vi "Camera Viewing Test.vi"() -> ()   [LabVIEW 2018]
uses:
  Classes/Realsense Cam/Private/Stream Config STYP.ctl
  Classes/Realsense Cam/Private/Stream Types Enum STYP.ctl
  Classes/Video Cam Processor/Video Cam Processor.lvclass
  C:/Users/aaron.jencks/Documents/GitHub/emerson_seed_object_detection/LabVIEW/Projects/Paul's Video Viewer/Classes/Realsense Cam Video File Wrapper/Realsense Cam File Wrapper.lvclass
  Classes/Realsense Cam/Realsense Cam.lvclass
panel:
  out "Roughness (inches)":T1
  out "spreadsheet string":string
  in  "Data Collection Interval (ms)":u32=10000
  in  "Next":bool
  out "Roughness":T1
  in  "Segmentedness":i32=10
  out "Image":T2(plugin-control)
  in  "stop":bool
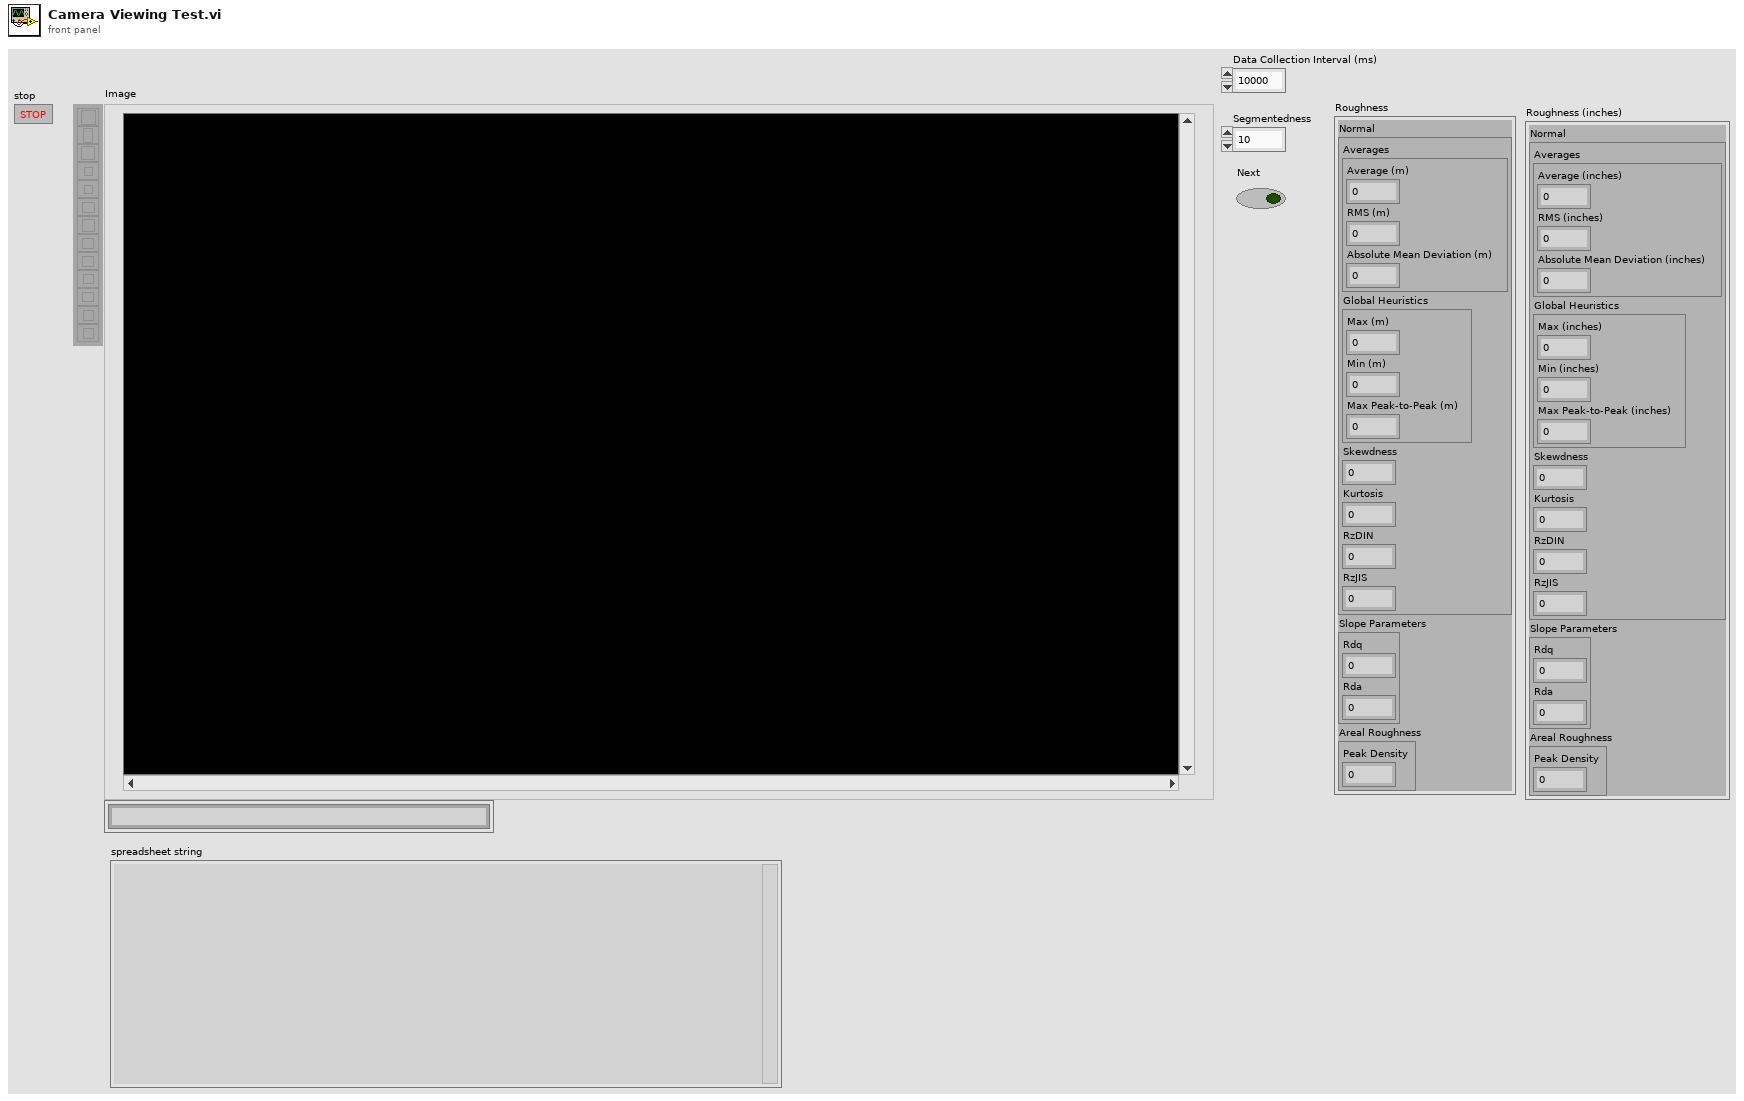
[diagram p1: front panel]
types:
  T1 = cluster{"Normal":cluster{"Averages":cluster{"Average":dbl, "RMS":dbl, "Absolute Mean Deviation":dbl}, "Global Heuristics":cluster{"Max":dbl, "Min":dbl, "Max Peak-to-Peak":dbl}, "Skewdness":dbl, "Kurtosis":dbl, "RzDIN":dbl, "RzJIS":dbl}, "Slope Parameters":cluster{"Rdq":dbl, "Rda":dbl}, "Areal Roughness":cluster{"Peak Density":dbl}}
  T2 = typedef "IMAQ Image.ctl" = refnum<image>
  T3 = cluster{"Normal":cluster{"Averages":cluster{"Average":dbl, "RMS":dbl, "Absolute Mean Deviation":dbl}, "Global Heuristics":cluster{"Max":dbl, "Min":dbl, "Max Peak-to-Peak":dbl}, "Skewdness":dbl, "Kurtosis":dbl, "RzDIN":dbl, "RzJIS":dbl}, "Slope Parameters":cluster{"Rdq":dbl, "Rda":dbl}, "Areal Roughness":cluster{"Peak Density":dbl}}[]
  T4 = typedef "Image Type" = u32
  T5 = typedef "Realsense Cam.lvclass/Stream Config STYP.ctl" = cluster{"Stream Type":T6, "Resolution":u16}
  T6 = typedef "Realsense Cam.lvclass/Stream Types Enum STYP.ctl" = enum16{"Depth", "Left IR", "Left IR Unrectified", "Right IR", "Right IR Unrectified", "Color", "RGB Ext."}
  T7 = cluster{"Average":dbl, "RMS":dbl, "Absolute Mean Deviation":dbl}
  T8 = cluster{"Max":dbl, "Min":dbl, "Max Peak-to-Peak":dbl}
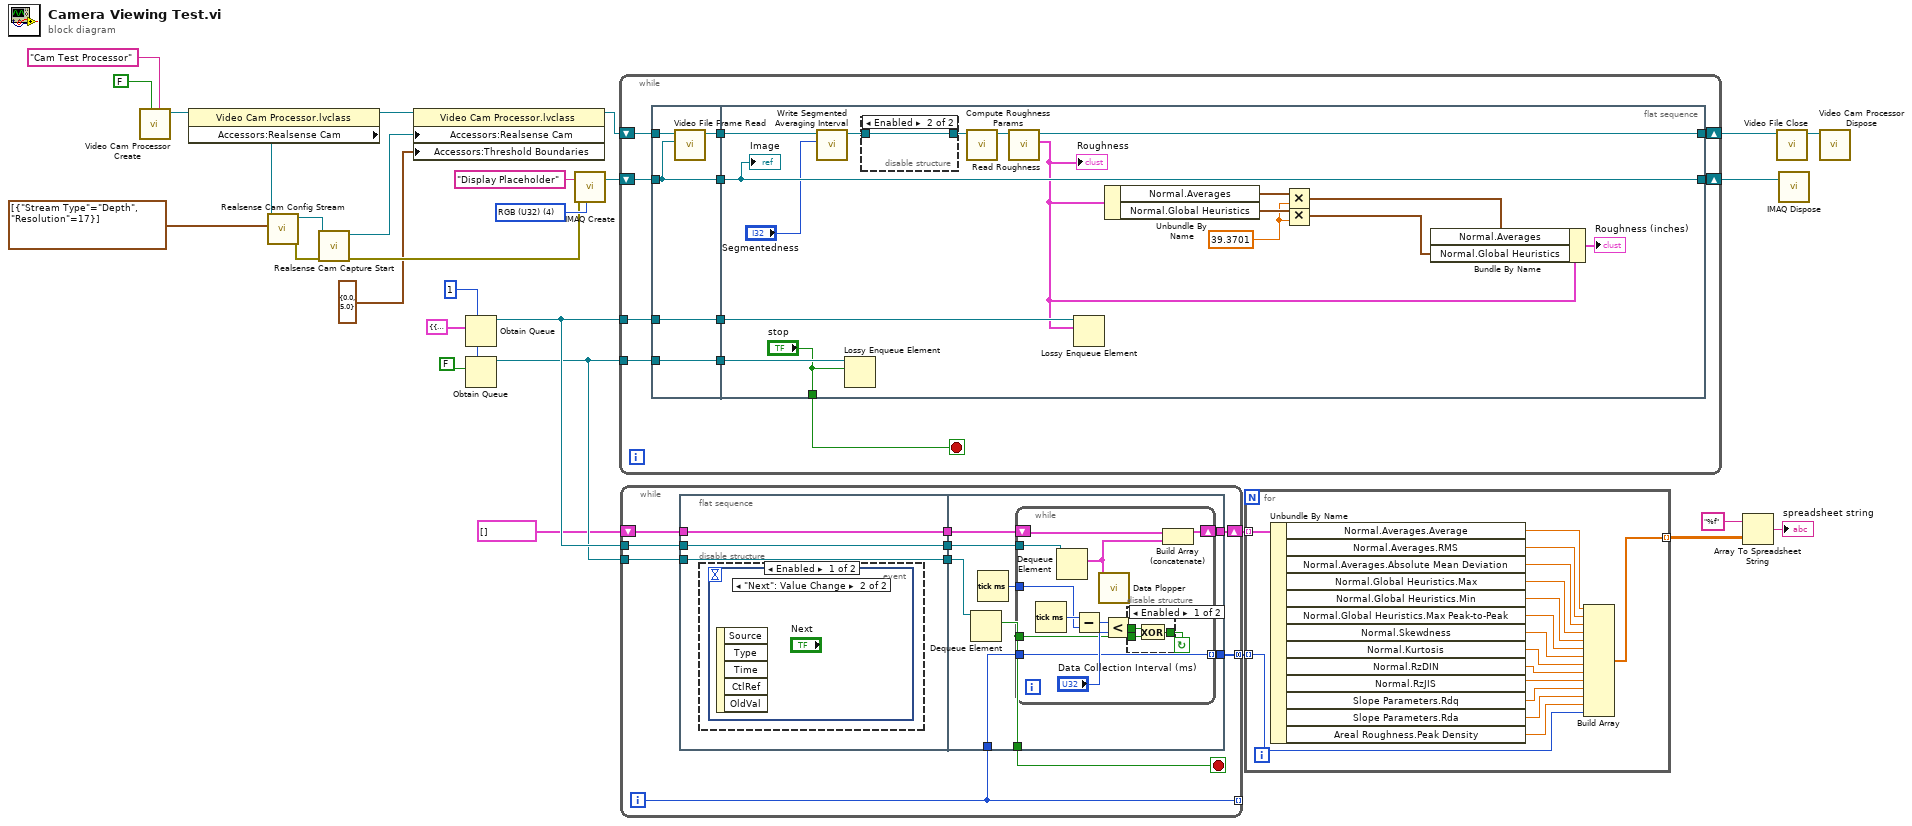
[diagram p0: block diagram]
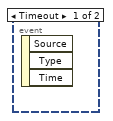
[diagram p2: hidden frame]
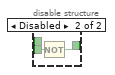
[diagram p4: hidden frame]
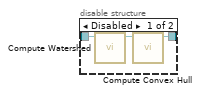
[diagram p5: hidden frame]
diagram:
  w8 = 1 ("max queue size (-1, unlimited)")
  w19 = T4 4 items=["Grayscale (U8)", "Grayscale (I16)", "Grayscale (SGL)", "Complex (CSG)", "RGB (U32)", "HSL (U32)", "RGB (U64)", "Grayscale (U16)"] ("Image Type")
  n1 = call "Video Cam Processor Create.vi"("Identifier"="Cam Test Processor", "Open? (T)"=FALSE) -> ("Video Processor out"=w26:refnum<class "Video Cam Processor.lvclass">)  [unwired: 8 in, 1 out]
  n2 = property class="Video Cam Processor.lvclass"(reference=w26) -> (reference out=w23:refnum<class "Video Cam Processor.lvclass">, "Accessors:Realsense Cam"=w25:refnum<class "Realsense Cam.lvclass">)  [unwired: 1 in, 1 out]
  n3 = call-dynamic "Realsense Cam Config Stream.vi"("Streams"=T5[] [{"Stream Type"=enum."Depth", "Resolution"=17}], "Realsense Cam in"=w25) -> ("error out"=w27:errorcluster, "Realsense Cam out"=w28:refnum<class "Realsense Cam.lvclass">)  [unwired: 8 in]
  n4 = call-dynamic "Realsense Cam Capture Start.vi"("error in (no error)"=w27, "Realsense Cam in"=w28) -> ("error out"=w15:errorcluster, "Realsense Cam out"=w22:refnum<class "Realsense Cam.lvclass">)  [unwired: 7 in, 1 out]
  n5 = property class="Video Cam Processor.lvclass"(reference=w23, "Accessors:Realsense Cam"=w22, "Accessors:Threshold Boundaries"=cluster{"Minimum":dbl, "Maximum":dbl} {"Minimum"=0.0, "Maximum"=5.0} ("Threshold Boundaries")) -> (reference out=w21:refnum<class "Video Cam Processor.lvclass">)  [unwired: 1 in, 1 out]
  n6 = Obtain Queue(max queue size (-1, unlimited)=w8, element data type=T1 {"Normal"={"Averages"={"Average"=0.671229863462704, "RMS"=0.6717750470164096, "Absolute Mean Deviation"=0.021225813170475925}, "Global Heuristics"={"Max"=0.7260000109672546, "Min"=0.5840000510215759, "Max Peak-to-Peak"=0.1419999599456787}, "Skewdness"=-0.6388644413310609, "Kurtosis"=3.710076081875204, "RzDIN"=0.08539999127388001, "RzJIS"=0.09479998350143433}, "Slope Parameters"={"Rdq"=0.002162500852052632, "Rda"=0.00044544842653668665}, "Areal Roughness"={"Peak Density"=0.0}} ("Roughness 2")) -> (queue out=w10:refnum<queue>)  [unwired: 3 in, 2 out]
  n7 = Obtain Queue(max queue size (-1, unlimited)=w8, element data type=FALSE) -> (queue out=w7:refnum<queue>)  [unwired: 3 in, 2 out]
  n8 = call "IMAQ Create"("Image Name"="Display Placeholder", "Image Type"=w19, "error in (no error)"=w15) -> ("New Image"=w18:T2)  [unwired: 2 in, 1 out]
  n9 = while {
    shift-right: [w39] -> w17
    shift-left: w21 -> [w40]
    shift-right: [w35] -> w16
    shift-left: w18 -> [w37]
    tunnel: w10 -> [w33]
    tunnel: w7 -> [w31]
    stop <- w30 stop-if-true
    n10 = flat-sequence {
      tunnel: w40 -> [w45]
      tunnel: w37 -> [w43]
      tunnel: [w44] -> w38
      tunnel: [w43] -> w36
      tunnel: [w42] -> w34
      tunnel: w33 -> [w42]
      tunnel: [w41] -> w32
      tunnel: w31 -> [w41]
      tunnel: [w59] -> w39
      tunnel: w38 -> [w61]
      tunnel: w36 -> [w62]
      tunnel: [w62] -> w35
      tunnel: w34 -> [w55]
      tunnel: w32 -> [w54]
      tunnel: ["stop"] -> w30
      frame #0 {
        n11 = call-dynamic "Video File Frame Read.vi"("Image Dst"=w43, "Video Processor in"=w45) -> ("Video Processor out"=w44:refnum<class "Video Cam Processor.lvclass">)  [unwired: 5 in, 4 out]
      }
      frame #1 {
        w49 = 39.3701
        n12 = call-dynamic "Write Segmented Averaging Interval.vi"("Segmented Averaging Interval"="Segmentedness", "Video Cam Processor in"=w61) -> ("Video Cam Processor out"=w58:refnum<class "Video Cam Processor.lvclass">)  [unwired: 8 in, 1 out]
        n13 = Lossy Enqueue Element(queue=w54, element="stop") -> ()  [unwired: 1 in, 4 out]
        n14 = disable-structure shown="Enabled" {
          disable-tunnel: w58 -> [w65 w66]
          disable-tunnel: [w63 w66] -> w57
          frame Disabled {
            n15 = call-dynamic "Compute Watershed.vi"("Video Cam Processor in"=w65) -> ("Video Cam Processor out"=w64:refnum<class "Video Cam Processor.lvclass">)  [unwired: 8 in, 2 out]
            n16 = call-dynamic "Compute Convex Hull.vi"("Video Cam Processor in"=w64) -> ("Video Cam Processor out"=w63:refnum<class "Video Cam Processor.lvclass">)  [unwired: 9 in, 1 out]
          }
          frame Enabled {
          }
        }
        n17 = call-dynamic "Compute Roughness Params.vi"("Video Cam Processor in"=w57) -> ("Video Cam Processor out"=w56:refnum<class "Video Cam Processor.lvclass">)  [unwired: 9 in, 1 out]
        n18 = call-dynamic "Read Roughness.vi"("Video Cam Processor in"=w56) -> ("Roughness"=w52:T1, "Video Cam Processor out"=w59:refnum<class "Video Cam Processor.lvclass">)  [unwired: 8 in, 1 out]
        "Roughness" <- w52
        n19 = Lossy Enqueue Element(queue=w55, element=w52) -> ()  [unwired: 1 in, 4 out]
        n20 = Unbundle By Name(w52) -> ("Normal.Averages"=w51:T7, "Normal.Global Heuristics"=w50:T8)
        n21 = Multiply(x=w51, y=w49) -> (x*y=w48:T7)
        n22 = Multiply(x=w50, y=w49) -> (x*y=w47:T8)
        n23 = Bundle By Name(cluster=w52, "Normal.Averages"=w48, "Normal.Global Heuristics"=w47) -> (→"Roughness (inches)":T1)
        "Image" <- w62
      }
    }
  }
  n24 = while {
    tunnel: w10 -> [w75]
    tunnel: w7 -> [w74]
    shift-right: [w69] -> w5
    shift-left: T3 [] -> [w70]
    tunnel: [w68] -> _ mode=indexing
    tunnel: [w67] -> w1 mode=concatenating
    i -> [w68]
    stop <- w72 stop-if-true
    n25 = flat-sequence {
      tunnel: [w79] -> w76
      tunnel: w75 -> [w79]
      tunnel: w74 -> [w78]
      tunnel: [w78] -> w73
      tunnel: [w77] -> w71
      tunnel: w70 -> [w77]
      tunnel: w76 -> [w87]
      tunnel: w73 -> [w86]
      tunnel: [w82] -> w72
      tunnel: w71 -> [w84]
      tunnel: [w83] -> w69
      tunnel: w68 -> [w81]
      tunnel: [w80] -> w67
      frame #0 {
        n26 = disable-structure shown="Enabled" {
          frame Enabled {
            n27 = event shown="[1] \"Next\": Value Change" {
              selector: _ -> [_ _]
              dyn-events: _ -> [_ _]
              timeout: _ -> [_ _]
              event Timeout {
                n28 = event-data() -> ()  [unwired: 1 in, 3 out]
              }
              event "Next": Value Change {
                n29 = event-data() -> ()  [unwired: 1 in, 5 out]
              }
            }
          }
          frame Disabled {
          }
        }
      }
      frame #1 {
        n30 = Dequeue Element(queue=w86) -> (element=w82:bool)  [unwired: 2 in, 3 out]
        n31 = Tick Count (ms)() -> (millisecond timer value=w85:u32)
        n32 = while {
          tunnel: w87 -> [w99]
          tunnel: w85 -> [w97]
          shift-right: [w94] -> w83
          shift-left: w84 -> [w93]
          tunnel: w82 -> [w89]
          tunnel: w81 -> [w88]
          tunnel: [w88] -> w80 mode=indexing
          stop <- w90 continue-if-true
          n33 = Tick Count (ms)() -> (millisecond timer value=w98:u32)
          n34 = Dequeue Element(queue=w99) -> (element=w92:T1)  [unwired: 2 in, 3 out]
          n35 = Subtract(x=w98, y=w97) -> (x-y=w96:u32)
          n36 = call "Data Plopper.vi"("Roughness"=w92) -> ()  [unwired: 11 in]
          n37 = Less?(x=w96, y="Data Collection Interval (ms)") -> (x < y?=w91:bool)
          n38 = disable-structure shown="Enabled" {
            disable-tunnel: w91 -> [w102 _]
            disable-tunnel: [w101 w103] -> w90
            disable-tunnel: w89 -> [w100 w104]
            frame Enabled {
              n39 = Exclusive Or(1:w100, 2:w102) -> (0:w101:bool)
            }
            frame Disabled {
              n40 = Not(x=w104) -> (.not. x?=w103:bool)
            }
          }
          n41 = Build Array (concatenate)(w93, w92) -> (w94:T3)
        }
      }
    }
  }
  n42 = for {
    tunnel: w5 -> [w120] mode=indexing
    tunnel: [w107] -> w4 mode=indexing
    tunnel: w1 -> [w106] mode=indexing
    n43 = Unbundle By Name(w120) -> ("Normal.Averages.Average"=w119:dbl, "Normal.Averages.RMS"=w118:dbl, "Normal.Averages.Absolute Mean Deviation"=w117:dbl, "Normal.Global Heuristics.Max"=w116:dbl, "Normal.Global Heuristics.Min"=w115:dbl, "Normal.Global Heuristics.Max Peak-to-Peak"=w114:dbl, "Normal.Skewdness"=w113:dbl, "Normal.Kurtosis"=w112:dbl, "Normal.RzDIN"=w111:dbl, "Normal.RzJIS"=w110:dbl, "Slope Parameters.Rdq"=w109:dbl, "Slope Parameters.Rda"=w108:dbl, "Areal Roughness.Peak Density"=w105:dbl)
    n44 = Build Array(w119, w118, w117, w116, w115, w114, w113, w112, w111, w110, w109, w108, w105, w106) -> (w107:dbl[])
  }
  n45 = Array To Spreadsheet String(array=w4, 3:"%f" ("format string")) -> (spreadsheet string=→"spreadsheet string":string)  [unwired: 1 in]
  n46 = call-dynamic "Video File Close.vi"("Realsense Cam File Wrapper in"=w17) -> ("Realsense Cam File Wrapper out"=w13:refnum<class "Video Cam Processor.lvclass">)  [unwired: 9 in, 1 out]
  n47 = call "IMAQ Dispose"("Image"=w16) -> ()  [unwired: 5 in, 1 out]
  n48 = call-dynamic "Video Cam Processor Dispose.vi"("Video Cam Processor in"=w13) -> ()  [unwired: 9 in, 2 out]
